vi "Display Channel Names (En Only).vi"(10 "Data Cluster":T1, 11 "16 EEG Channels":T4(array[cluster])) -> (2 "En MAP":u16)   [LabVIEW 2019, in "CML UI.lvlib"]
doc: "This VI Updates Only enabled channel's names from selected Montage"
uses:
  CML UI.lvlib
  Module Data--cluster.ctl
  Acquisition State.ctl
  Measurement UI Displays.ctl
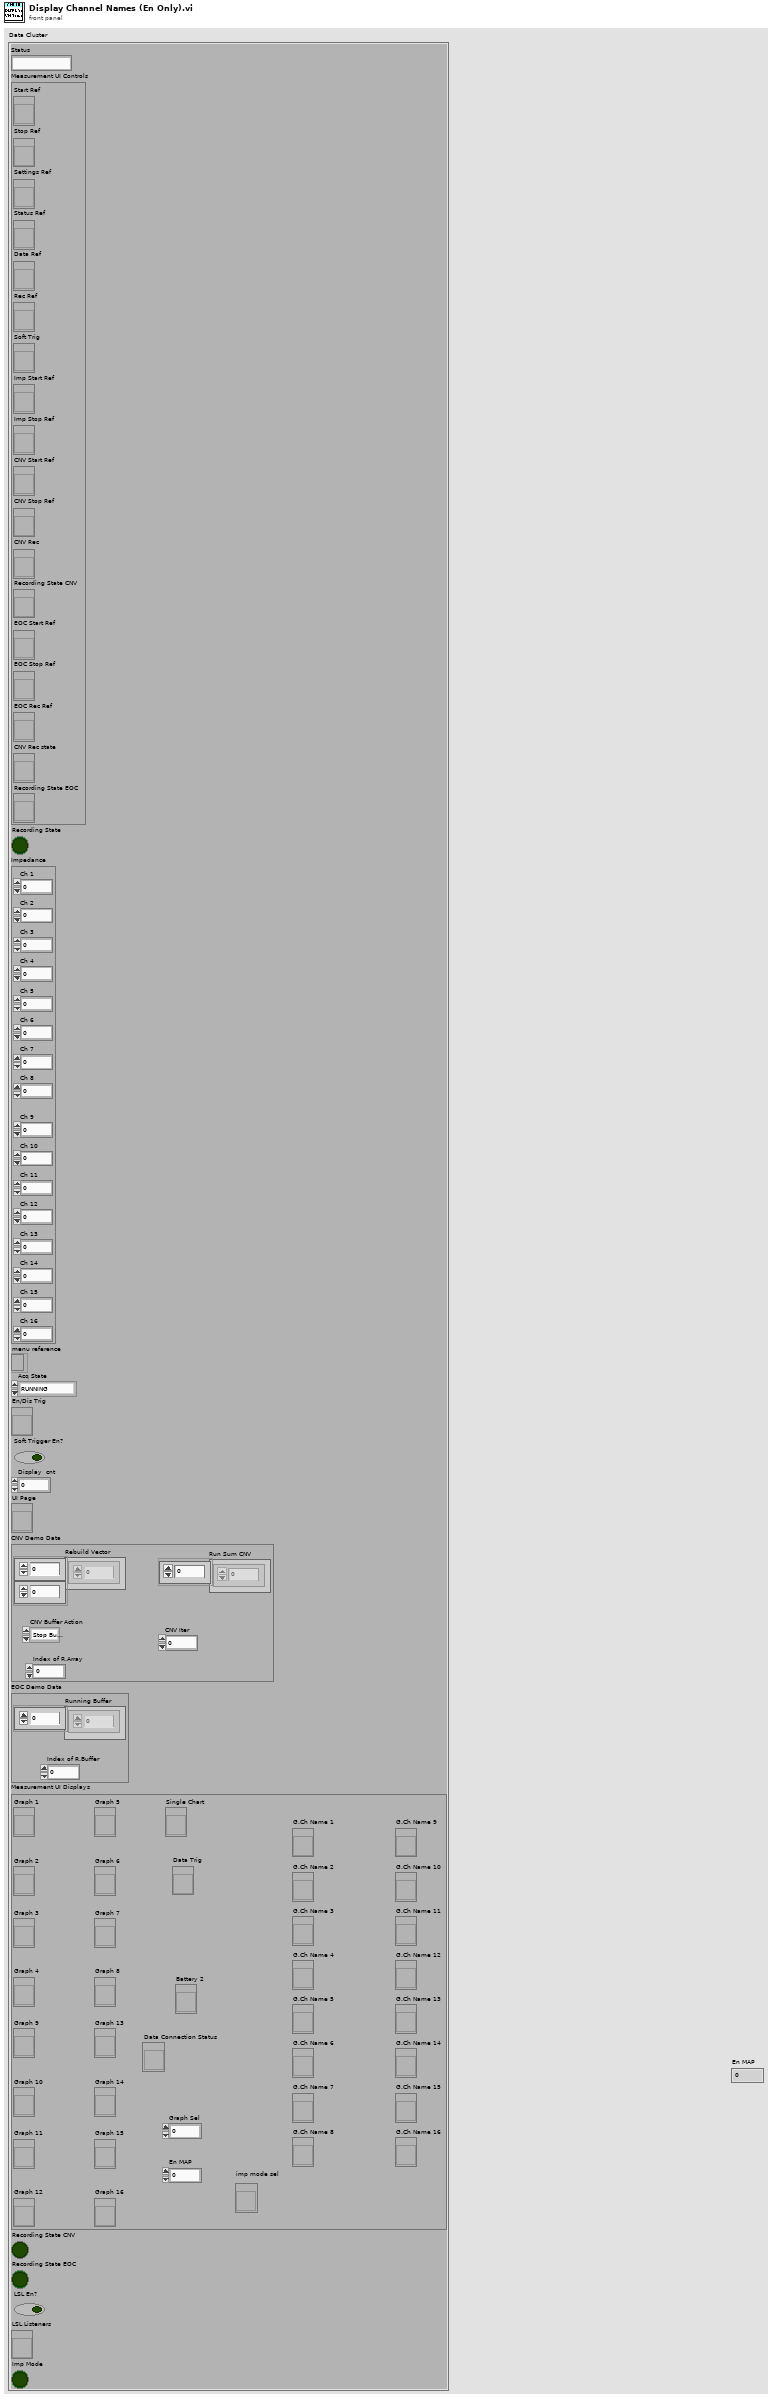
[diagram p1: front panel]
types:
  T1 = typedef "CML UI.lvlib/Module Data--cluster.ctl" = cluster{"Status":string, "Measurement UI Controls":cluster{"Start Ref":refnum<vi>, "Stop Ref":refnum<vi>, "Settings Ref":refnum<vi>, "Status Ref":refnum<vi>, "Data Ref":refnum<vi>, "Rec Ref":refnum<vi>, "Soft Trig":refnum<vi>, "Imp Start Ref":refnum<vi>, "Imp Stop Ref":refnum<vi>, "CNV Start Ref":refnum<vi>, "CNV Stop Ref":refnum<vi>, "CNV Rec":refnum<vi>, "Recording State CNV":refnum<vi>, "EOC Start Ref":refnum<vi>, "EOC Stop Ref":refnum<vi>, "EOC Rec Ref":refnum<vi>, "CNV Rec state":refnum<vi>, "Recording State EOC":refnum<vi>}, "Recording State":bool, "Impedance":cluster{"Ch 1":dbl, "Ch 2":dbl, "Ch 3":dbl, "Ch 4":dbl, "Ch 5":dbl, "Ch 6":dbl, "Ch 7":dbl, "Ch 8":dbl, "Ch 9":dbl, "Ch 10":dbl, "Ch 11":dbl, "Ch 12":dbl, "Ch 13":dbl, "Ch 14":dbl, "Ch 15":dbl, "Ch 16":dbl}, "menu reference ":refnum<k9>, "Acq State":T2, "En/Dis Trig":refnum<vi>, "Soft Trigger En?":bool, "Display  cnt":u8, "UI Page":refnum<vi>, "CNV Demo Data":cluster{"Rebuild Vector":dbl[][], "CNV Buffer Action":enum16{"Stop Buffer Fill", "Start Buffer Fill", "Analyze Buffer"}, "Index of R.Array":u16, "Run Sum CNV":dbl[], "CNV Iter":u16}, "EOC Demo Data":cluster{"Running Buffer":dbl[], "Index of R.Buffer":u8}, "Measurement UI Displays":T3, "Recording State CNV":bool, "Recording State EOC":bool, "LSL En?":bool, "LSL Listeners":refnum<vi>, "Imp Mode":bool}
  T2 = typedef "CML UI.lvlib/Acquisition State.ctl" = enum16{"RUNNING", "IDLE"}
  T3 = typedef "CML UI.lvlib/Measurement UI Displays.ctl" = cluster{"Graph 1":refnum<vi>, "Graph 2":refnum<vi>, "Graph 3":refnum<vi>, "Graph 4":refnum<vi>, "Graph 5":refnum<vi>, "Graph 6":refnum<vi>, "Graph 7":refnum<vi>, "Graph 8":refnum<vi>, "Graph 9":refnum<vi>, "Graph 10":refnum<vi>, "Graph 11":refnum<vi>, "Graph 12":refnum<vi>, "Graph 13":refnum<vi>, "Graph 14":refnum<vi>, "Graph 15":refnum<vi>, "Graph 16":refnum<vi>, "Battery 2":refnum<vi>, "Data Trig":refnum<vi>, "Data Connection Status":refnum<vi>, "Graph Sel":u8, "En MAP":u16, "Single Chart":refnum<vi>, "G.Ch Name 1":refnum<vi>, "G.Ch Name 2":refnum<vi>, "G.Ch Name 3":refnum<vi>, "G.Ch Name 4":refnum<vi>, "G.Ch Name 5":refnum<vi>, "G.Ch Name 6":refnum<vi>, "G.Ch Name 7":refnum<vi>, "G.Ch Name 8":refnum<vi>, "G.Ch Name 9":refnum<vi>, "G.Ch Name 10":refnum<vi>, "G.Ch Name 11":refnum<vi>, "G.Ch Name 12":refnum<vi>, "G.Ch Name 13":refnum<vi>, "G.Ch Name 14":refnum<vi>, "G.Ch Name 15":refnum<vi>, "G.Ch Name 16":refnum<vi>, "imp mode sel":refnum<vi>}
  T4 = cluster{"Channel Name":string, "Channel No":u8, "Channel Enabled":bool, "Channel Referenced":bool}[]
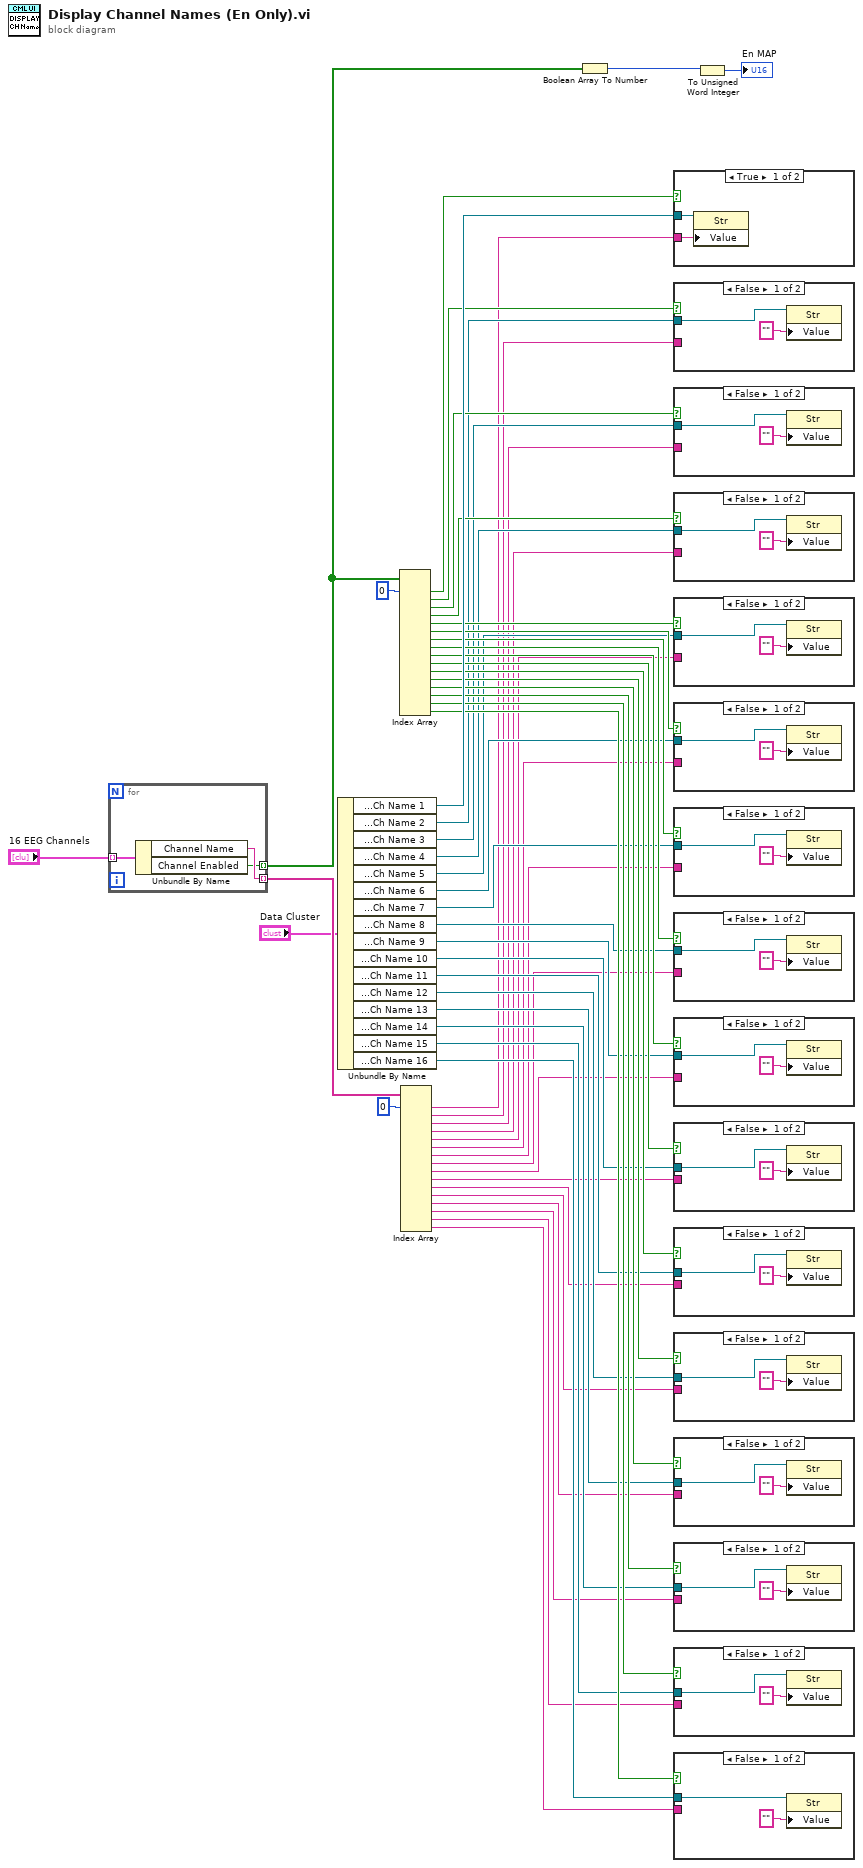
[diagram p0: block diagram]
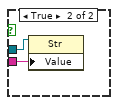
[diagram p2: hidden frame]
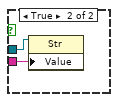
[diagram p3: hidden frame]
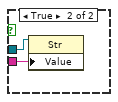
[diagram p4: hidden frame]
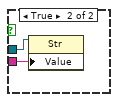
[diagram p5: hidden frame]
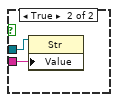
[diagram p6: hidden frame]
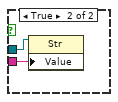
[diagram p7: hidden frame]
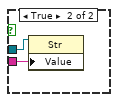
[diagram p8: hidden frame]
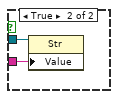
[diagram p9: hidden frame]
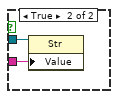
[diagram p10: hidden frame]
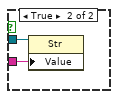
[diagram p11: hidden frame]
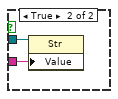
[diagram p12: hidden frame]
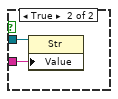
[diagram p13: hidden frame]
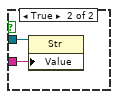
[diagram p14: hidden frame]
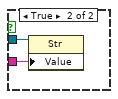
[diagram p15: hidden frame]
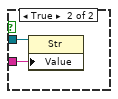
[diagram p16: hidden frame]
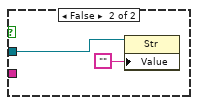
[diagram p17: hidden frame]
diagram:
  n1 = for {
    tunnel: "16 EEG Channels" -> [w59] mode=indexing
    tunnel: [w58] -> w55 mode=indexing
    tunnel: [w57] -> w3 mode=indexing
    n2 = Unbundle By Name(w59) -> ("Channel Name"=w58:string, "Channel Enabled"=w57:bool)
  }
  n3 = Unbundle By Name("Data Cluster") -> ("Measurement UI Displays.G.Ch Name 1"=w52:refnum<vi>, "Measurement UI Displays.G.Ch Name 2"=w34:refnum<vi>, "Measurement UI Displays.G.Ch Name 3"=w33:refnum<vi>, "Measurement UI Displays.G.Ch Name 4"=w32:refnum<vi>, "Measurement UI Displays.G.Ch Name 5"=w31:refnum<vi>, "Measurement UI Displays.G.Ch Name 6"=w30:refnum<vi>, "Measurement UI Displays.G.Ch Name 7"=w29:refnum<vi>, "Measurement UI Displays.G.Ch Name 8"=w28:refnum<vi>, "Measurement UI Displays.G.Ch Name 9"=w27:refnum<vi>, "Measurement UI Displays.G.Ch Name 10"=w26:refnum<vi>, "Measurement UI Displays.G.Ch Name 11"=w25:refnum<vi>, "Measurement UI Displays.G.Ch Name 12"=w24:refnum<vi>, "Measurement UI Displays.G.Ch Name 13"=w23:refnum<vi>, "Measurement UI Displays.G.Ch Name 14"=w22:refnum<vi>, "Measurement UI Displays.G.Ch Name 15"=w21:refnum<vi>, "Measurement UI Displays.G.Ch Name 16"=w20:refnum<vi>)
  n4 = Index Array(array=w3, index #1=0 ("index")) -> (element #1=w50:bool, element #2=w49:bool, element #3=w48:bool, element #4=w47:bool, element #5=w46:bool, element #6=w45:bool, element #7=w44:bool, element #8=w43:bool, element #9=w42:bool, element #10=w41:bool, element #11=w40:bool, element #12=w39:bool, element #13=w38:bool, element #14=w37:bool, element #15=w36:bool, element #16=w35:bool)  [unwired: 15 in]
  n5 = Index Array(array=w55, index #1=0 ("index")) -> (element #1=w19:string, element #2=w18:string, element #3=w17:string, element #4=w16:string, element #5=w15:string, element #6=w14:string, element #7=w13:string, element #8=w12:string, element #9=w11:string, element #10=w10:string, element #11=w9:string, element #12=w8:string, element #13=w7:string, element #14=w6:string, element #15=w5:string, element #16=w4:string)  [unwired: 15 in]
  n6 = Boolean Array To Number(Boolean array=w3) -> (number=w2:u32)
  n7 = case shown="True" w50 {
    tunnel: w52 -> [w61 w63]
    tunnel: w19 -> [w60 _]
    frame True {
      n8 = property class="Str"(reference=w61, "Value"=w60) -> ()  [unwired: 1 in, 2 out]
    }
    frame False {
      n9 = property class="Str"(reference=w63, "Value"="") -> ()  [unwired: 1 in, 2 out]
    }
  }
  n10 = case shown="False" w49 {
    tunnel: w34 -> [w65 w67]
    tunnel: w18 -> [_ w66]
    frame False {
      n11 = property class="Str"(reference=w65, "Value"="") -> ()  [unwired: 1 in, 2 out]
    }
    frame True {
      n12 = property class="Str"(reference=w67, "Value"=w66) -> ()  [unwired: 1 in, 2 out]
    }
  }
  n13 = case shown="False" w48 {
    tunnel: w33 -> [w69 w71]
    tunnel: w17 -> [_ w70]
    frame False {
      n14 = property class="Str"(reference=w69, "Value"="") -> ()  [unwired: 1 in, 2 out]
    }
    frame True {
      n15 = property class="Str"(reference=w71, "Value"=w70) -> ()  [unwired: 1 in, 2 out]
    }
  }
  n16 = case shown="False" w47 {
    tunnel: w32 -> [w73 w75]
    tunnel: w16 -> [_ w74]
    frame False {
      n17 = property class="Str"(reference=w73, "Value"="") -> ()  [unwired: 1 in, 2 out]
    }
    frame True {
      n18 = property class="Str"(reference=w75, "Value"=w74) -> ()  [unwired: 1 in, 2 out]
    }
  }
  n19 = case shown="False" w46 {
    tunnel: w31 -> [w77 w79]
    tunnel: w15 -> [_ w78]
    frame False {
      n20 = property class="Str"(reference=w77, "Value"="") -> ()  [unwired: 1 in, 2 out]
    }
    frame True {
      n21 = property class="Str"(reference=w79, "Value"=w78) -> ()  [unwired: 1 in, 2 out]
    }
  }
  n22 = case shown="False" w45 {
    tunnel: w30 -> [w81 w83]
    tunnel: w14 -> [_ w82]
    frame False {
      n23 = property class="Str"(reference=w81, "Value"="") -> ()  [unwired: 1 in, 2 out]
    }
    frame True {
      n24 = property class="Str"(reference=w83, "Value"=w82) -> ()  [unwired: 1 in, 2 out]
    }
  }
  n25 = case shown="False" w44 {
    tunnel: w29 -> [w85 w87]
    tunnel: w13 -> [_ w86]
    frame False {
      n26 = property class="Str"(reference=w85, "Value"="") -> ()  [unwired: 1 in, 2 out]
    }
    frame True {
      n27 = property class="Str"(reference=w87, "Value"=w86) -> ()  [unwired: 1 in, 2 out]
    }
  }
  n28 = case shown="False" w43 {
    tunnel: w28 -> [w89 w91]
    tunnel: w12 -> [_ w90]
    frame False {
      n29 = property class="Str"(reference=w89, "Value"="") -> ()  [unwired: 1 in, 2 out]
    }
    frame True {
      n30 = property class="Str"(reference=w91, "Value"=w90) -> ()  [unwired: 1 in, 2 out]
    }
  }
  n31 = case shown="False" w42 {
    tunnel: w27 -> [w93 w95]
    tunnel: w11 -> [_ w94]
    frame False {
      n32 = property class="Str"(reference=w93, "Value"="") -> ()  [unwired: 1 in, 2 out]
    }
    frame True {
      n33 = property class="Str"(reference=w95, "Value"=w94) -> ()  [unwired: 1 in, 2 out]
    }
  }
  n34 = case shown="False" w41 {
    tunnel: w26 -> [w97 w99]
    tunnel: w10 -> [_ w98]
    frame False {
      n35 = property class="Str"(reference=w97, "Value"="") -> ()  [unwired: 1 in, 2 out]
    }
    frame True {
      n36 = property class="Str"(reference=w99, "Value"=w98) -> ()  [unwired: 1 in, 2 out]
    }
  }
  n37 = case shown="False" w40 {
    tunnel: w25 -> [w101 w103]
    tunnel: w9 -> [_ w102]
    frame False {
      n38 = property class="Str"(reference=w101, "Value"="") -> ()  [unwired: 1 in, 2 out]
    }
    frame True {
      n39 = property class="Str"(reference=w103, "Value"=w102) -> ()  [unwired: 1 in, 2 out]
    }
  }
  n40 = case shown="False" w39 {
    tunnel: w24 -> [w105 w107]
    tunnel: w8 -> [_ w106]
    frame False {
      n41 = property class="Str"(reference=w105, "Value"="") -> ()  [unwired: 1 in, 2 out]
    }
    frame True {
      n42 = property class="Str"(reference=w107, "Value"=w106) -> ()  [unwired: 1 in, 2 out]
    }
  }
  n43 = case shown="False" w38 {
    tunnel: w23 -> [w109 w111]
    tunnel: w7 -> [_ w110]
    frame False {
      n44 = property class="Str"(reference=w109, "Value"="") -> ()  [unwired: 1 in, 2 out]
    }
    frame True {
      n45 = property class="Str"(reference=w111, "Value"=w110) -> ()  [unwired: 1 in, 2 out]
    }
  }
  n46 = case shown="False" w37 {
    tunnel: w22 -> [w113 w115]
    tunnel: w6 -> [_ w114]
    frame False {
      n47 = property class="Str"(reference=w113, "Value"="") -> ()  [unwired: 1 in, 2 out]
    }
    frame True {
      n48 = property class="Str"(reference=w115, "Value"=w114) -> ()  [unwired: 1 in, 2 out]
    }
  }
  n49 = case shown="False" w36 {
    tunnel: w21 -> [w117 w119]
    tunnel: w5 -> [_ w118]
    frame False {
      n50 = property class="Str"(reference=w117, "Value"="") -> ()  [unwired: 1 in, 2 out]
    }
    frame True {
      n51 = property class="Str"(reference=w119, "Value"=w118) -> ()  [unwired: 1 in, 2 out]
    }
  }
  n52 = case shown="False" w35 {
    tunnel: w20 -> [w121 w123]
    tunnel: w4 -> [_ w122]
    frame False {
      n53 = property class="Str"(reference=w121, "Value"="") -> ()  [unwired: 1 in, 2 out]
    }
    frame True {
      n54 = property class="Str"(reference=w123, "Value"=w122) -> ()  [unwired: 1 in, 2 out]
    }
  }
  n55 = To Unsigned Word Integer(number=w2) -> (unsigned 16bit integer=→"En MAP":u16)
